vi "stats.vi"(8 "error in (no error)":errorcluster, 10 "actuatorout":dbl, 11 "RSA in":refnum<class "RSA.lvclass">) -> (0 "error out":errorcluster, 1 "actuatorout 2":dbl, 2 "Array":dbl[](array[numeric]), 3 "RSA out":refnum<class "RSA.lvclass">)   [LabVIEW 2012, in "RSA.lvclass"]
uses:
  RSA.lvclass
  RSA.lvclass/RSA.ctl
panel:
  out "size(s)":i32
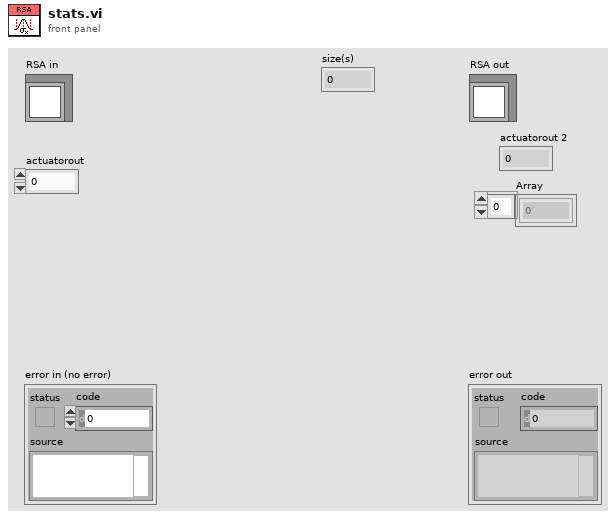
[diagram p1: front panel]
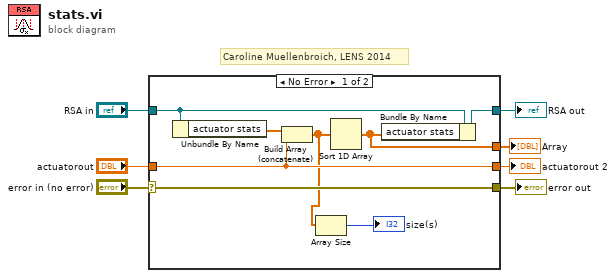
[diagram p0: block diagram]
diagram:
  # "Caroline Muellenbroich, LENS 2014"
  n1 = case shown="No Error" "error in (no error)" {
    selector: "error in (no error)" -> [w15 w18]
    tunnel: [w15 w18] -> w6
    tunnel: [w13 w17] -> w4
    tunnel: "RSA in" -> [w14 w17]
    tunnel: "actuatorout" -> [w10 w16]
    tunnel: [w10 w16] -> w2
    tunnel: [w12 _] -> w1
    frame No Error {
      n2 = Unbundle By Name(w14) -> ("actuator stats"=w11:dbl[])
      n3 = Build Array (concatenate)(w11, w10) -> (w9:dbl[])
      n4 = Array Size(array=w9) -> (size(s)=→"size(s)":i32)
      n5 = Sort 1D Array(array=w9) -> (sorted array=w12:dbl[])
      n6 = Bundle By Name(cluster=w14, "actuator stats"=w12) -> (w13:refnum<class "RSA.lvclass">)
    }
    frame Error {
    }
  }
  "error out" <- w6
  "RSA out" <- w4
  "actuatorout 2" <- w2
  "Array" <- w1
